vi "target.vi"() -> ()   [LabVIEW 2014]
uses:
  <vilib>/Platform/TimedLoop/XDataNode/timing_clust.ctl
  <vilib>/Platform/TimedLoop/XDataNode/nitl_modes.ctl
  <vilib>/Platform/TimedLoop/XDataNode/wakeup.ctl
  states.ctl
  <vilib>/rvi/FXPMathLib/FxpConvert/subVIs/nifxpmath_Convert_SimConfig.ctl
  <vilib>/fxp/LVFixedPointQuantizationPolicyTypeDef.ctl
  <vilib>/fxp/LVFixedPointOverflowPolicyTypeDef.ctl
  <vilib>/rvi/FXPMathLib/SharedSubVIs/typedef/nifxpmath_BASIC_ImplementationSettings.ctl
  <vilib>/rvi/Emulation/niFpgaGetClockAttributes.vi
  <vilib>/rvi/Emulation/niFpgaSctlEmulationGetInTimedLoop.vi
  <vilib>/rvi/Emulation/niFpgaEmulationReportErrorSimple.vi
  <vilib>/rvi/Emulation/niFpgaEmulationIsFPGAContextNoSignature.vi
  <vilib>/rvi/errors/niFpgaSetErrorForExecOnDevCompSimple.vi
  <vilib>/rvi/eio/common/nirviEmuReportErrorAndStop.vi
  <vilib>/rvi/DataTransferAndStorage/Container/Common/niFpgaContainerGetUniqueNameForEmu.vi
  <vilib>/rvi/FIFO/Fifo_Resource/nirvififoEmulationSetSize.vi
  <vilib>/rvi/FIFO/Fifo_Resource/nirviFifoEmulationQueueMgr.vi
  <instcachedir>/0/nirviFifoEmulationQueueMgr_E5CAEC123FF24DC58D834DCA3CDAA9B5.lvgen/nirviFifoEmulationQueueMgr_E5CAEC123FF24DC58D834DCA3CDAA9B5_003.vi
  <vilib>/rvi/FIFO/Fifo_Resource/nirvififoEmulationCreateLock.vi
  <vilib>/rvi/Emulation/niFpgaProcessEmulError.vi
  <vilib>/rvi/FIFO/Fifo_Resource/nirvififoEmulationObtainLock.vi
  <vilib>/rvi/FIFO/Fifo_Resource/nirvififoEmulationReleaseLock.vi
  <vilib>/rvi/occurrence/nirviWaitOnOccurrenceBase.vi
  <vilib>/rvi/errors/nirviReportUnexpectedCaseInternalError.vi
  <vilib>/rvi/errors/nirviReportUnexpectedCaseInternalError (U32).vi
  <vilib>/rvi/eio/common/nirviEmuTemplateMethod_errors.vi
  <vilib>/rvi/interface/RandomDataEmulation/niFpgaRandomDataHandleErrors.vi
  <vilib>/rvi/Emulation/niFpgaCriticalErrorInLSC.vi
  <instcachedir>/0/nirviFifoEmulationQueueMgr_E5CAEC123FF24DC58D834DCA3CDAA9B5.lvgen/nirviFifoEmulationQueueMgr_E5CAEC123FF24DC58D834DCA3CDAA9B5_019.vi
  <vilib>/rvi/Memory/Memory_Emulation/nirvimemoryFastEmulation.vi
  <vilib>/rvi/Memory/Memory_Emulation/nirvimemoryEmulation.vi
  <vilib>/rvi/FIFO/Fifo_Resource/nirvififoEmulationDetermineInputValidOut.vi
  <vilib>/rvi/FXPMathLib/FxpConvert/simVIs/DllFxpConvertTemp_sub.vi
  <vilib>/rvi/ClientSDK/Core/DevComputerLib/Private/FourWireProtocol(cint64).vi
  <instcachedir>/0/nirviFifoEmulationQueueMgr_E5CAEC123FF24DC58D834DCA3CDAA9B5.lvgen/nirviFifoEmulationQueueMgr_E5CAEC123FF24DC58D834DCA3CDAA9B5_011.vi
  <vilib>/rvi/DataTransferAndStorage/Container/XNode/niFpgaContainer.xnode
  <vilib>/rvi/FIFO/Fifo_Resource/nirvififoEmulationRead.vi
  <vilib>/eio/EIONode/EIONode.xnode
  <vilib>/rvi/interface/RandomDataEmulation/nirviRandomDataFpgaReadWriteTemplate.vi
  <vilib>/Platform/TimedLoop/XDataNode/XDataNode.xnode
  <vilib>/rvi/FIFO/Fifo_Resource/nirvififoEmulationWrite.vi
  <vilib>/rvi/FXPMathLib/FxpConvert/XNode/nifxpmath_Convert.xnode
  <vilib>/rvi/FXPMathLib/FxpMultComplex/XNode/niFpgaMultComplex.xnode
  <vilib>/rvi/ClientSDK/Core/DevComputerLib/niFpgaDevCompUtilities.lvlib
  <vilib>/Platform/TimedLoop/XDataNode/XDNodeRunTimeDep.lvlib
panel:
  out "transfer ticks":u32
  in  "noise":bool
  out "data timeout":bool
  out "rx":fxp<+/-,12,1>
  out "tx ticks":u32
  out "tx":i16
  out "signal":i8
  out "acquisition ticks":u32
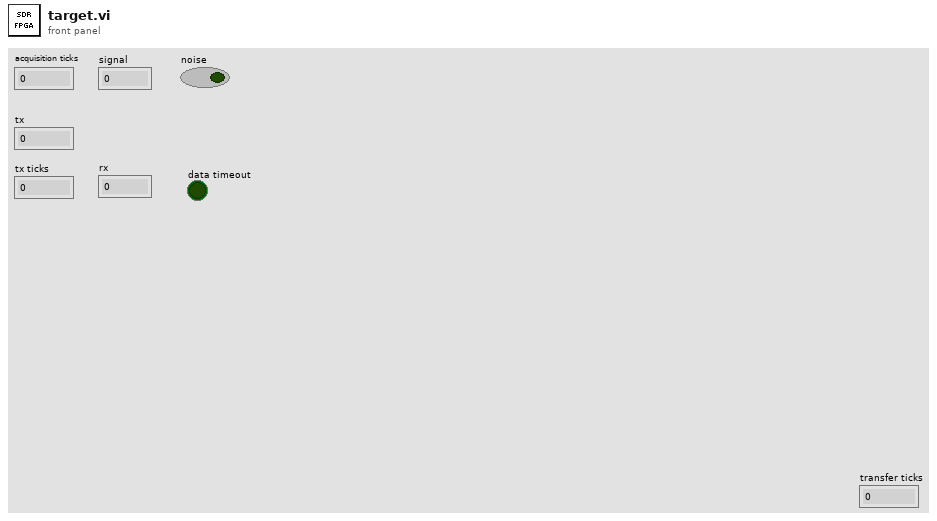
[diagram p1: front panel]
types:
  T1 = typedef "XDNodeRunTimeDep.lvlib/timing_clust.ctl" = cluster{"Expected End [f-1]":u64, "Actual End [f-1]":u64, "Finished Late? [f-1]":bool, "Expected End [i-1]":u64, "Actual End [i-1]":u64, "Finished Late? [i-1]":bool, "Expected Start [i]":u64, "Actual Start [i]":u64, "Expected Start [f]":u64, "Actual Start [f]":u64, "Source Name":string, "Structure Name":string, "Period":i64, "Deadline":i64, "Offset":i64, "Start":i64, "Priority":i32, "Timeout":i32, "Mode":T2, "Wakeup Reason":T3, "Error":errorcluster, "Source Type":string, "Secondary Source Type":string, "Global End Time":u64, "Global Start Time":u64, "Frame Duration":u64, "Iteration Duration":u64, "Assigned CPU":i32, "I/O Scan Engine Mode":u32}
  T2 = typedef "XDNodeRunTimeDep.lvlib/nitl_modes.ctl" = enum32{"No Change", "Process missed periods, maintain original phase", "Discard missed periods, maintain original phase", "Process missed periods, ignore original phase", "Discard missed periods, ignore original phase"}
  T3 = typedef "XDNodeRunTimeDep.lvlib/wakeup.ctl" = enum32{"Normal", "Aborted", "Asynchronous wakeup", "Timing source error", "Timed loop error", "Timeout"}
  T4 = typedef "states.ctl" = enum16{"read sample", "write zero", "hold", "wait"}
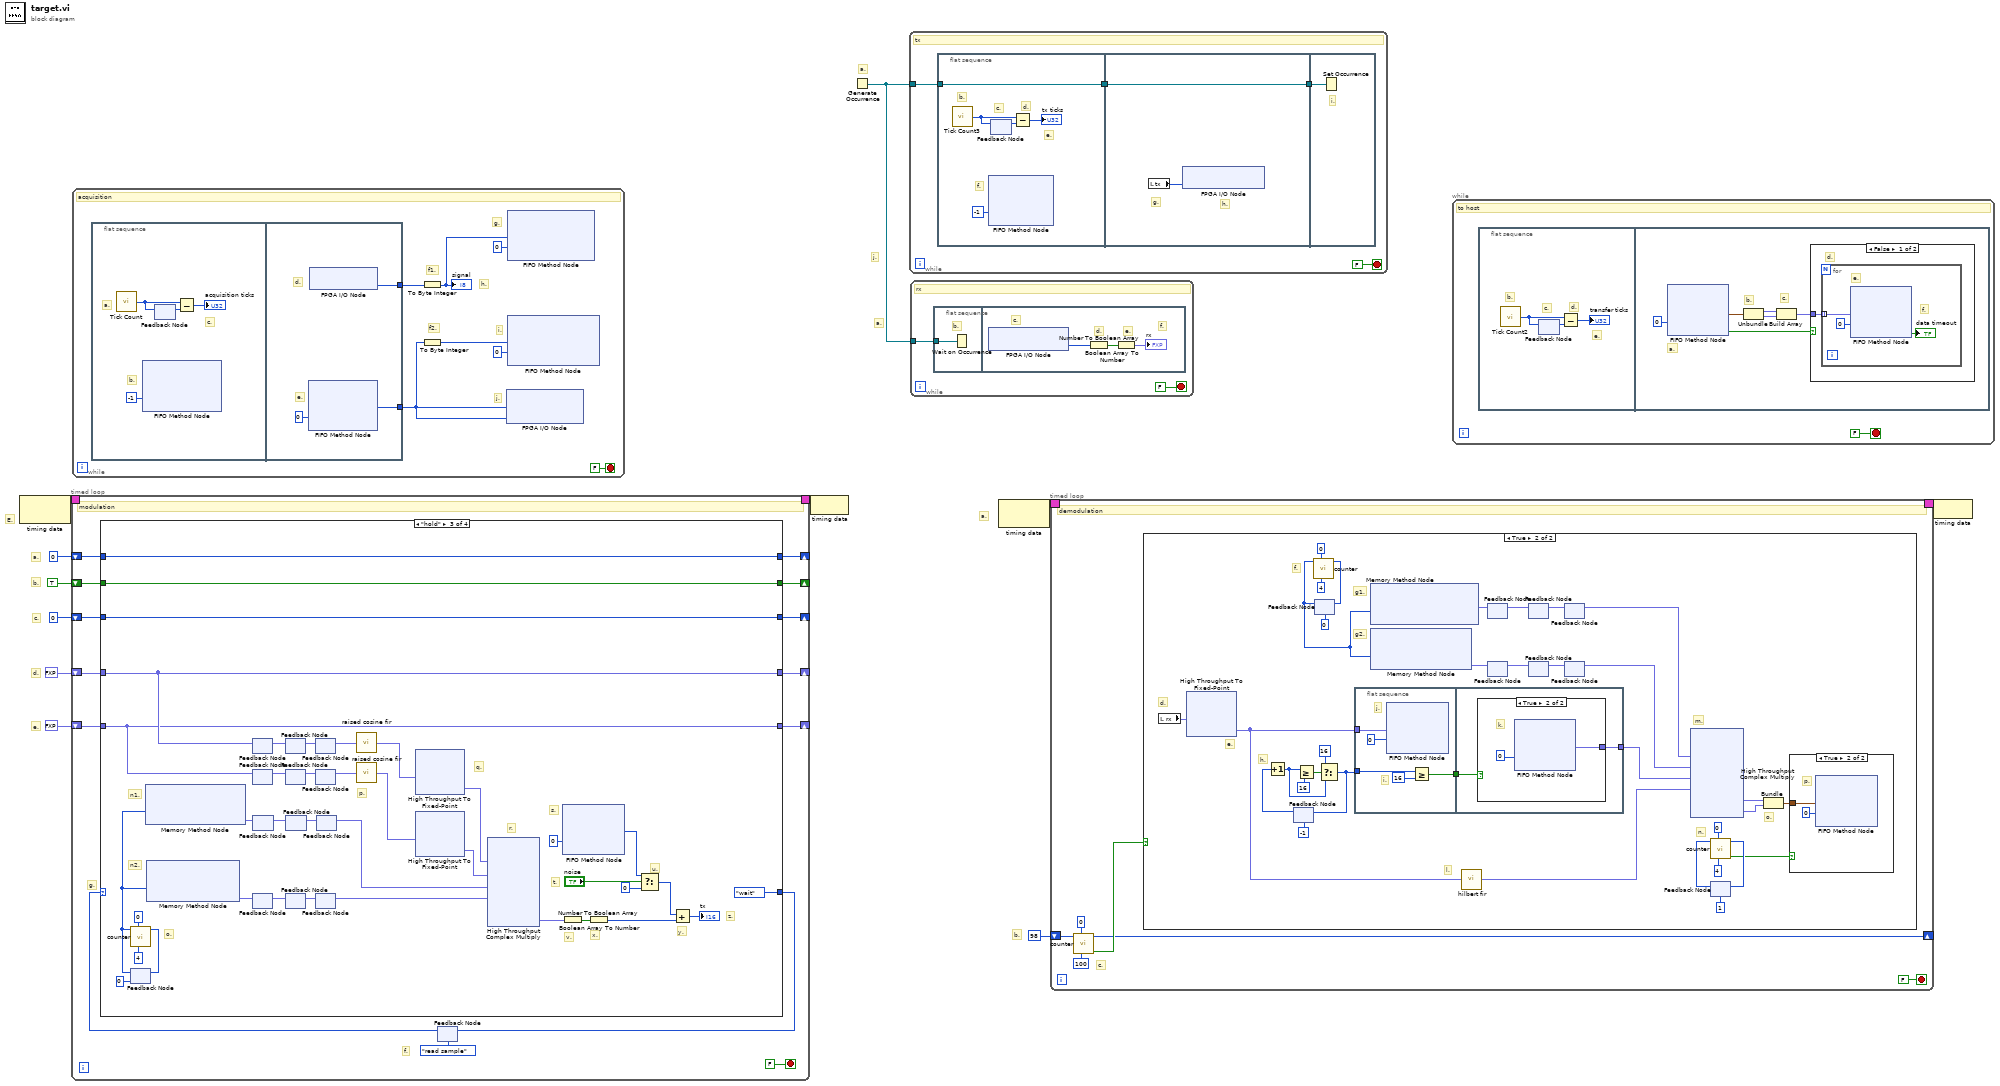
[diagram p0: block diagram]
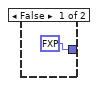
[diagram p5: hidden frame]
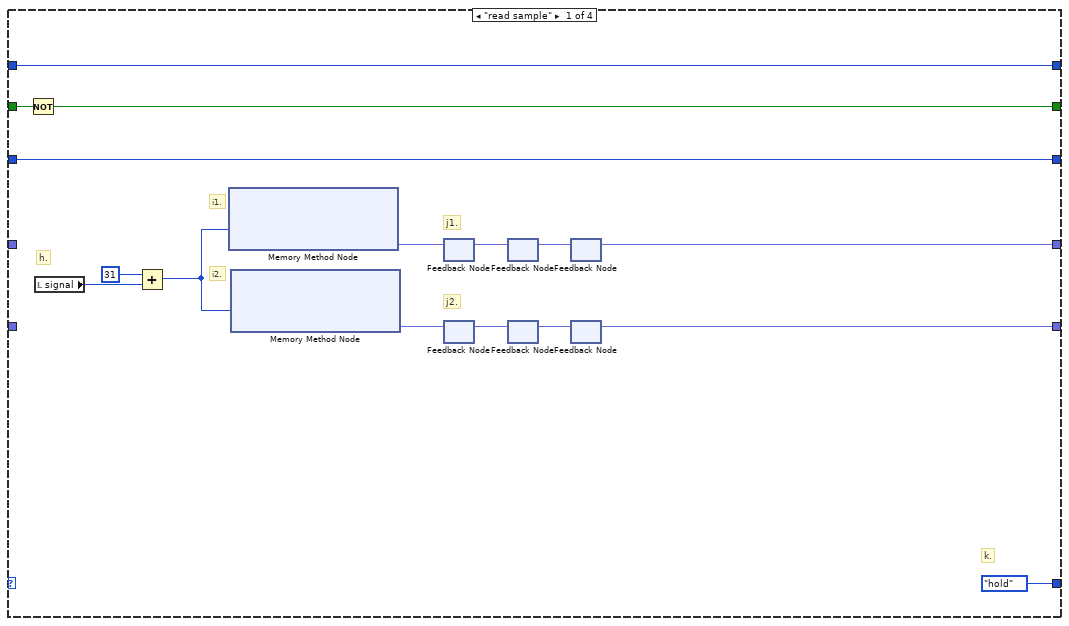
[diagram p6: hidden frame]
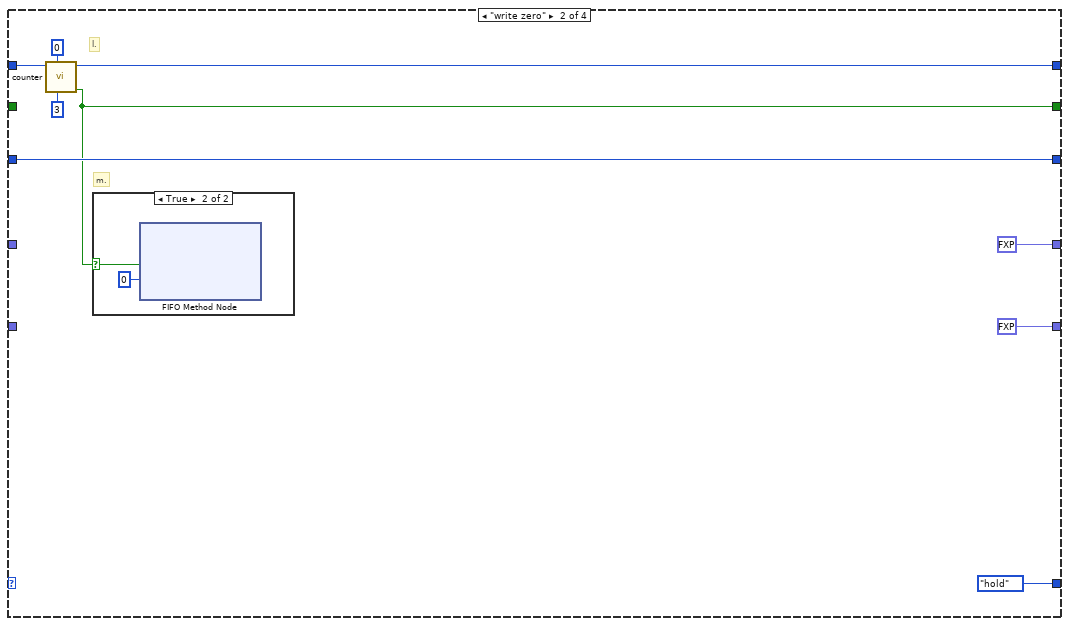
[diagram p7: hidden frame]
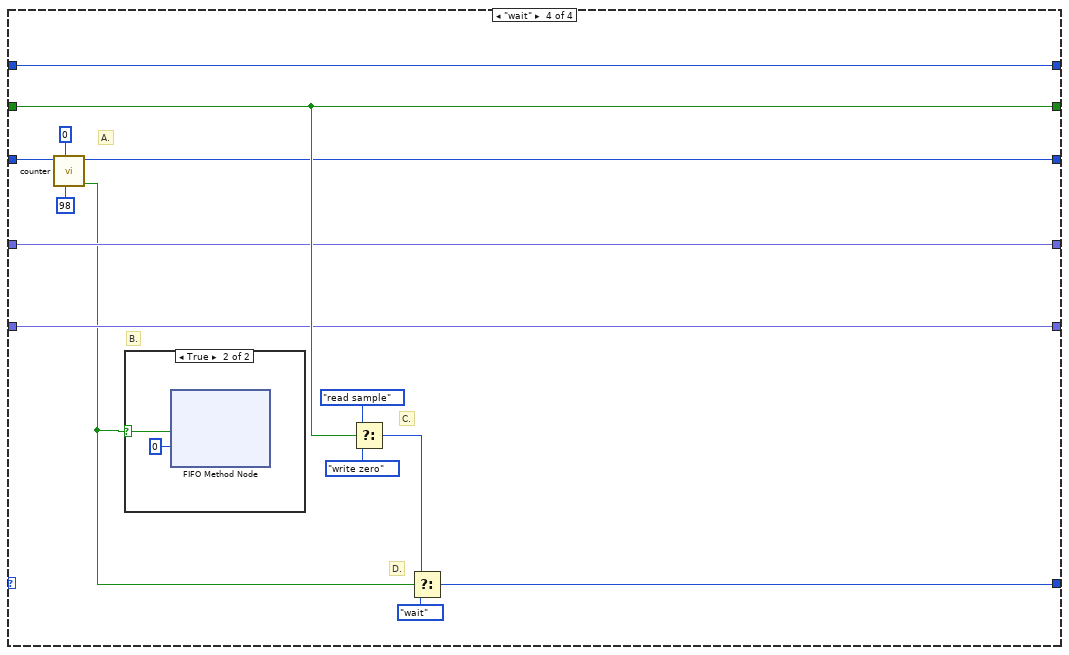
[diagram p9: hidden frame]
diagram:
  # "b."
  # "a."
  # "a."
  # "j."
  # "a."
  # "E."
  # "e."
  # "d."
  # "c."
  # "b."
  # "a."
  n1 = node-c288() -> (w11:T1)  [unwired: 1 in]
  n2 = timed-loop {
    shift-right: [w21] -> _
    shift-left: i16 0 -> [w22]
    shift-right: [w19] -> _
    shift-left: i16 0 -> [w20]
    shift-right: [w18] -> _
    shift-left: TRUE -> [w17]
    timing: w11 -> [_]
    timing-out: [_] -> w10
    shift-right: [w16] -> _
    shift-left: fxp<+/-,16,1> 0.0 ("Data") -> [w14]
    shift-right: [w15] -> _
    shift-left: fxp<+/-,16,1> 0.0 ("Data") -> [w13]
    stop <- FALSE stop-if-true
    # "g."
    # "f."
    # "modulation"
    n3 = feedback #1(states."read sample" ("Enum")) -> (w25:T4)
    n4 = case shown="\"hold\"" w25 {
      tunnel: [states."hold" ("Enum") states."hold" ("Enum") states."wait" ("Enum") w264] -> w24
      tunnel: w22 -> [w40 w46 w89 w260]
      tunnel: [w40 w43 w89 w260] -> w21
      tunnel: w20 -> [w39 w49 w87 w256]
      tunnel: [w39 w49 w87 w254] -> w19
      tunnel: [w37 w42 w88 w259] -> w18
      tunnel: w17 -> [w38 _ w88 w259]
      tunnel: [w30 fxp<+/-,16,1> 0.0 ("Data") w75 w258] -> w16
      tunnel: [w29 fxp<+/-,16,1> 0.0 ("Data") w74 w257] -> w15
      tunnel: w14 -> [_ _ w75 w258]
      tunnel: w13 -> [_ _ w74 w257]
      frame "read sample" {
        # "j2."
        # "i2."
        # "k."
        # "j1."
        # "i1."
        # "h."
        n5 = Not(x=w38) -> (.not. x?=w37:bool)
        n6 = local read "signal"() -> (w31:i8)
        n7 = Add(x=i8 31, y=w31) -> (x+y=w28:i8)
        n8 = xnode ("Memory Method Node")("Address"=w28) -> ("Data"=w27:fxp<+/-,16,1>)  [unwired: 1 in, 1 out]
        n9 = xnode ("Memory Method Node")("Address"=w28) -> ("Data"=w26:fxp<+/-,16,1>)  [unwired: 1 in, 1 out]
        n10 = feedback #2() -> (w35:fxp<+/-,16,1>)  [unwired: 1 in]
        n11 = feedback-in #2(w27) -> ()
        n12 = feedback #3() -> (w34:fxp<+/-,16,1>)  [unwired: 1 in]
        n13 = feedback-in #3(w26) -> ()
        n14 = feedback #4() -> (w36:fxp<+/-,16,1>)  [unwired: 1 in]
        n15 = feedback-in #4(w35) -> ()
        n16 = feedback #5() -> (w33:fxp<+/-,16,1>)  [unwired: 1 in]
        n17 = feedback-in #5(w34) -> ()
        n18 = feedback #6() -> (w30:fxp<+/-,16,1>)  [unwired: 1 in]
        n19 = feedback-in #6(w36) -> ()
        n20 = feedback #7() -> (w29:fxp<+/-,16,1>)  [unwired: 1 in]
        n21 = feedback-in #7(w33) -> ()
      }
      frame "write zero" {
        # "m."
        # "l."
        n22 = call "counter.vi"("final"=i16 3, "reset"=i16 0, "counter in"=w46) -> ("trigger"=w42:bool, "counter out"=w43:i16)  [unwired: 7 in]
        n23 = case shown="True" w42 {
          selector: w42 -> [_ w52]
          frame False {
          }
          frame True {
            n24 = xnode ("FIFO Method Node")("Element"=w52, "Timeout"=0) -> ()  [unwired: 1 in, 2 out]
          }
        }
      }
      frame "hold" {
        # "z."
        # "y."
        # "x."
        # "v."
        # "u."
        # "t."
        # "s."
        # "r."
        # "q."
        # "n2."
        # "p."
        # "o."
        # "n1."
        n25 = feedback #8(i16 0) -> (w71:i16)
        n26 = call "counter.vi"("final"=i16 4 ("y"), "reset"=i16 0 ("t"), "counter in"=w71) -> ("counter out"=w68:i16)  [unwired: 7 in, 1 out]
        n27 = feedback-in #8(w68) -> ()
        n28 = xnode ("Memory Method Node")("Address"=w71) -> ("Data"=w85:fxp<+/-,2,2>)  [unwired: 1 in, 1 out]
        n29 = xnode ("Memory Method Node")("Address"=w71) -> ("Data"=w86:fxp<+/-,2,2>)  [unwired: 1 in, 1 out]
        n30 = feedback #9() -> (w78:fxp<+/-,16,1>)  [unwired: 1 in]
        n31 = feedback-in #9(w75) -> ()
        n32 = feedback #10() -> (w77:fxp<+/-,16,1>)  [unwired: 1 in]
        n33 = feedback-in #10(w74) -> ()
        n34 = feedback #11() -> (w82:fxp<+/-,2,2>)  [unwired: 1 in]
        n35 = feedback-in #11(w86) -> ()
        n36 = feedback #12() -> (w83:fxp<+/-,2,2>)  [unwired: 1 in]
        n37 = feedback-in #12(w85) -> ()
        n38 = feedback #13() -> (w79:fxp<+/-,16,1>)  [unwired: 1 in]
        n39 = feedback-in #13(w78) -> ()
        n40 = feedback #14() -> (w76:fxp<+/-,16,1>)  [unwired: 1 in]
        n41 = feedback-in #14(w77) -> ()
        n42 = feedback #15() -> (w81:fxp<+/-,2,2>)  [unwired: 1 in]
        n43 = feedback-in #15(w82) -> ()
        n44 = feedback #16() -> (w84:fxp<+/-,2,2>)  [unwired: 1 in]
        n45 = feedback-in #16(w83) -> ()
        n46 = feedback #17() -> (w73:fxp<+/-,16,1>)  [unwired: 1 in]
        n47 = feedback-in #17(w79) -> ()
        n48 = feedback #18() -> (w72:fxp<+/-,16,1>)  [unwired: 1 in]
        n49 = feedback-in #18(w76) -> ()
        n50 = feedback #19() -> (w64:fxp<+/-,2,2>)  [unwired: 1 in]
        n51 = feedback-in #19(w81) -> ()
        n52 = feedback #20() -> (w65:fxp<+/-,2,2>)  [unwired: 1 in]
        n53 = feedback-in #20(w84) -> ()
        n54 = call "raised cosine fir.vi"("data"=w73) -> ("filtered"=w67:fxp<+/-,19,2>)  [unwired: 4 in]
        n55 = call "raised cosine fir.vi"("data"=w72) -> ("filtered"=w66:fxp<+/-,19,2>)  [unwired: 4 in]
        n56 = xnode "High Throughput To Fixed-Point"("x"=w67) -> ("y"=w63:fxp<+/-,8,1>)
        n57 = xnode "High Throughput To Fixed-Point"("x"=w66) -> ("y"=w62:fxp<+/-,8,1>)
        n58 = xnode ("High Throughput Complex Multiply")("xr"=w63, "xi"=w62, "yr"=w65, "yi"=w64) -> ("pi"=w60:fxp<+/-,12,1>)  [unwired: 1 out]
        n59 = xnode ("FIFO Method Node")("Timeout"=0) -> ("Element"=w55:i16)  [unwired: 1 in, 2 out]
        n60 = Number To Boolean Array(number=w60) -> (Boolean array=w61:bool[])
        n61 = Boolean Array To Number(Boolean array=w61) -> (number=w59:i16)
        n62 = Select(t=w55, s="noise", f=i16 0) -> (s? t:f=w53:i16)
        n63 = Add(x=w53, y=w59) -> (x+y=→"tx":i16)
      }
      frame "wait" {
        # "D."
        # "C."
        # "B."
        # "A."
        n64 = call "counter.vi"("final"=i16 98 ("control"), "reset"=i16 0 ("y"), "counter in"=w256) -> ("trigger"=w252:bool, "counter out"=w254:i16)  [unwired: 7 in]
        n65 = case shown="True" w252 {
          selector: w252 -> [_ w267]
          frame False {
          }
          frame True {
            n66 = xnode ("FIFO Method Node")("Element"=w267, "Timeout"=0) -> ()  [unwired: 1 in, 2 out]
          }
        }
        n67 = Select(t=states."read sample" ("Enum"), s=w259, f=states."write zero" ("Enum")) -> (s? t:f=w261:T4)
        n68 = Select(t=w261, s=w252, f=states."wait" ("Enum")) -> (s? t:f=w264:T4)
      }
    }
    n69 = feedback-in #1(w24) -> ()
  }
  n70 = while {
    stop <- FALSE stop-if-true
    # "j."
    # "i."
    # "h."
    # "g."
    # "f2."
    # "f1."
    # "acquisition"
    n71 = flat-sequence {
      tunnel: [w283] -> w275
      tunnel: [w281] -> w273
      frame #0 {
        # "c."
        # "b."
        # "a."
        n72 = call "Tick Count"() -> ("Tick Count(Ticks)"=w279:u32)
        n73 = xnode ("FIFO Method Node")("Timeout"=-1) -> ()  [unwired: 1 in, 3 out]
        n74 = feedback-in #21(w279) -> ()
        n75 = feedback #21() -> (w280:u32)  [unwired: 1 in]
        n76 = Subtract(x=w279, y=w280) -> (x-y=→"acquisition ticks":u32)
      }
      frame #1 {
        # "e."
        # "d."
        n77 = xnode ("FIFO Method Node")("Timeout"=0) -> ("Element"=w281:i16)  [unwired: 1 in, 2 out]
        n78 = xnode "FPGA I/O Node"() -> ("AudioIn/Left"=w283:i16)  [unwired: 1 in, 1 out]
      }
    }
    n79 = To Byte Integer(number=w275) -> (8bit integer=w274:i8)
    "signal" <- w274
    n80 = To Byte Integer(number=w273) -> (8bit integer=w272:i8)
    n81 = xnode "FPGA I/O Node"("AudioOut/Left"=w273, "AudioOut/Right"=w273) -> ()  [unwired: 2 in, 2 out]
    n82 = xnode ("FIFO Method Node")("Element"=w274, "Timeout"=0) -> ()  [unwired: 1 in, 2 out]
    n83 = xnode ("FIFO Method Node")("Element"=w272, "Timeout"=0) -> ()  [unwired: 1 in, 2 out]
  }
  n84 = node-c288(w10) -> ()
  n85 = Generate Occurrence() -> (w1:refnum<k4>)
  n86 = while {
    tunnel: w1 -> [w284]
    stop <- FALSE stop-if-true
    # "tx"
    n87 = flat-sequence {
      tunnel: [w288] -> w285
      tunnel: w284 -> [w288]
      tunnel: [w294] -> w286
      tunnel: w285 -> [w294]
      tunnel: w286 -> [w295]
      frame #0 {
        # "f."
        # "e."
        # "d."
        # "c."
        # "b."
        n88 = call "Tick Count3"() -> ("Tick Count(Ticks)"=w291:u32)
        n89 = xnode ("FIFO Method Node")("Timeout"=-1) -> ()  [unwired: 1 in, 3 out]
        n90 = feedback #22() -> (w292:u32)  [unwired: 1 in]
        n91 = feedback-in #22(w291) -> ()
        n92 = Subtract(x=w291, y=w292) -> (x-y=→"tx ticks":u32)
      }
      frame #1 {
        # "h."
        # "g."
        n93 = local read "tx"() -> (w293:i16)
        n94 = xnode "FPGA I/O Node"("ConnectorC/AO0"=w293) -> ()  [unwired: 1 in, 1 out]
      }
      frame #2 {
        # "i."
        n95 = Set Occurrence(w295) -> ()
      }
    }
  }
  n96 = while {
    tunnel: w1 -> [w296]
    stop <- FALSE stop-if-true
    # "rx"
    n97 = flat-sequence {
      tunnel: w296 -> [w298]
      frame #0 {
        # "b."
        n98 = Wait on Occurrence(2:w298) -> ()  [unwired: 2 in, 1 out]
      }
      frame #1 {
        # "f."
        # "e."
        # "d."
        # "c."
        n99 = xnode "FPGA I/O Node"() -> ("ConnectorC/AI0"=w299:i16)  [unwired: 1 in, 1 out]
        n100 = Number To Boolean Array(number=w299) -> (Boolean array=w301:bool[])
        n101 = Boolean Array To Number(Boolean array=w301) -> (number=→"rx":fxp<+/-,12,1>)
      }
    }
  }
  n102 = node-c288() -> (w4:T1)  [unwired: 1 in]
  n103 = timed-loop {
    timing: w4 -> [_]
    timing-out: [_] -> w3
    shift-right: [w305] -> _
    shift-left: i16 98 ("counter initial") -> [w302]
    stop <- FALSE stop-if-true
    # "c."
    # "demodulation"
    n104 = call "counter.vi"("final"=i16 100, "reset"=i16 0 ("x"), "counter in"=w302) -> ("trigger"=w306:bool, "counter out"=w305:i16)  [unwired: 7 in]
    n105 = case shown="True" w306 {
      frame False {
      }
      frame True {
        # "o."
        # "n."
        # "m."
        # "l."
        # "h."
        # "g2."
        # "g1."
        # "f."
        # "e."
        # "d."
        n106 = local read "rx"() -> (w318:fxp<+/-,12,1>)
        n107 = xnode "High Throughput To Fixed-Point"("x"=w318) -> ("y"=w321:fxp<+/-,20,4>)
        n108 = feedback #23(-1) -> (w328:i32)
        n109 = Increment(x=w328) -> (x+1=w332:i32)
        n110 = Greater Or Equal?(x=w332, y=16 ("x")) -> (x >= y?=w330:bool)
        n111 = feedback #24(i16 0) -> (w308:i16)
        n112 = call "counter.vi"("final"=i16 4 ("y"), "reset"=i16 0 ("t"), "counter in"=w308) -> ("counter out"=w326:i16)  [unwired: 7 in, 1 out]
        n113 = feedback-in #24(w326) -> ()
        n114 = Select(t=16 ("x"), s=w330, f=w332) -> (s? t:f=w334:i32)
        n115 = feedback-in #23(w334) -> ()
        n116 = flat-sequence {
          tunnel: w321 -> [w484]
          tunnel: w334 -> [w487]
          tunnel: [w485] -> w327
          tunnel: [w489] -> w316
          tunnel: w327 -> [w488]
          frame #0 {
            # "j."
            # "i."
            n117 = xnode ("FIFO Method Node")("Element"=w484, "Timeout"=0) -> ()  [unwired: 1 in, 2 out]
            n118 = Greater Or Equal?(x=w487, y=16) -> (x >= y?=w485:bool)
          }
          frame #1 {
            n119 = case shown="True" w488 {
              tunnel: [fxp<+/-,20,4> 0.0 ("Element") w491] -> w489
              frame False {
              }
              frame True {
                # "k."
                n120 = xnode ("FIFO Method Node")("Timeout"=0) -> ("Element"=w491:fxp<+/-,20,4>)  [unwired: 1 in, 2 out]
              }
            }
          }
        }
        n121 = xnode ("Memory Method Node")("Address"=w308) -> ("Data"=w323:fxp<+/-,16,1>)  [unwired: 1 in, 1 out]
        n122 = xnode ("Memory Method Node")("Address"=w308) -> ("Data"=w322:fxp<+/-,16,1>)  [unwired: 1 in, 1 out]
        n123 = call "hilbert fir.vi"("x(n)"=w321) -> ("y(n)"=w315:fxp<+/-,20,4>)  [unwired: 4 in]
        n124 = feedback #25() -> (w336:fxp<+/-,16,1>)  [unwired: 1 in]
        n125 = feedback-in #25(w323) -> ()
        n126 = feedback #26() -> (w337:fxp<+/-,16,1>)  [unwired: 1 in]
        n127 = feedback-in #26(w322) -> ()
        n128 = feedback #27() -> (w335:fxp<+/-,16,1>)  [unwired: 1 in]
        n129 = feedback-in #27(w336) -> ()
        n130 = feedback #28() -> (w338:fxp<+/-,16,1>)  [unwired: 1 in]
        n131 = feedback-in #28(w337) -> ()
        n132 = feedback #29() -> (w339:fxp<+/-,16,1>)  [unwired: 1 in]
        n133 = feedback-in #29(w335) -> ()
        n134 = feedback #30() -> (w340:fxp<+/-,16,1>)  [unwired: 1 in]
        n135 = feedback-in #30(w338) -> ()
        n136 = xnode ("High Throughput Complex Multiply")("xr"=w339, "xi"=w340, "yr"=w316, "yi"=w315) -> ("pr"=w320:fxp<+/-,20,4>, "pi"=w319:fxp<+/-,20,4>)
        n137 = feedback #31(i16 1 ("counter out")) -> (w311:i16)
        n138 = call "counter.vi"("final"=i16 4, "reset"=i16 0 ("x"), "counter in"=w311) -> ("trigger"=w309:bool, "counter out"=w312:i16)  [unwired: 7 in]
        n139 = feedback-in #31(w312) -> ()
        n140 = Bundle("pr"=w320, "pi"=w319) -> (w317:cluster{"pr":fxp<+/-,20,4>, "pi":fxp<+/-,20,4>})  [unwired: 1 in]
        n141 = case shown="True" w309 {
          tunnel: w317 -> [_ w342]
          frame False {
          }
          frame True {
            # "p."
            n142 = xnode ("FIFO Method Node")("Element"=w342, "Timeout"=0) -> ()  [unwired: 1 in, 2 out]
          }
        }
      }
    }
  }
  n143 = while {
    stop <- FALSE stop-if-true
    # "to host"
    n144 = flat-sequence {
      frame #0 {
        # "e."
        # "d."
        # "c."
        # "b."
        n145 = call "Tick Count2"() -> ("Tick Count(Ticks)"=w497:u32)
        n146 = feedback #32() -> (w496:u32)  [unwired: 1 in]
        n147 = feedback-in #32(w497) -> ()
        n148 = Subtract(x=w497, y=w496) -> (x-y=→"transfer ticks":u32)
      }
      frame #1 {
        # "c."
        # "b."
        # "a."
        n149 = xnode ("FIFO Method Node")("Timeout"=0) -> ("Element"=w504:cluster{"pr":fxp<+/-,20,4>, "pi":fxp<+/-,20,4>}, "Timed Out?"=w499:bool)  [unwired: 1 in, 1 out]
        n150 = Unbundle(w504) -> ("pr"=w502:fxp<+/-,20,4>, "pi"=w501:fxp<+/-,20,4>)
        n151 = Build Array(w502, w501) -> (w500:fxp<+/-,20,4>[])
        n152 = case shown="False" w499 {
          tunnel: w500 -> [w505 _]
          frame False {
            # "d."
            n153 = for {
              tunnel: w505 -> [w508] mode=indexing
              # "f."
              # "e."
              n154 = xnode ("FIFO Method Node")("Element"=w508, "Timeout"=0) -> ("Timed Out?"=→"data timeout":bool)  [unwired: 1 in, 1 out]
            }
          }
          frame True {
          }
        }
      }
    }
  }
  n155 = node-c288(w3) -> ()
